vi "Terminal-GearSystem-Getter.vi"(8 "error in (no error)":errorcluster caption="错误输入（无错误）", 11 "read operation timeout (ms)":i32=5000 caption="读操作超时（5000毫秒）") -> (0 "error out":errorcluster caption="错误输出", 3 "设备信息":T1)   [LabVIEW 2014]
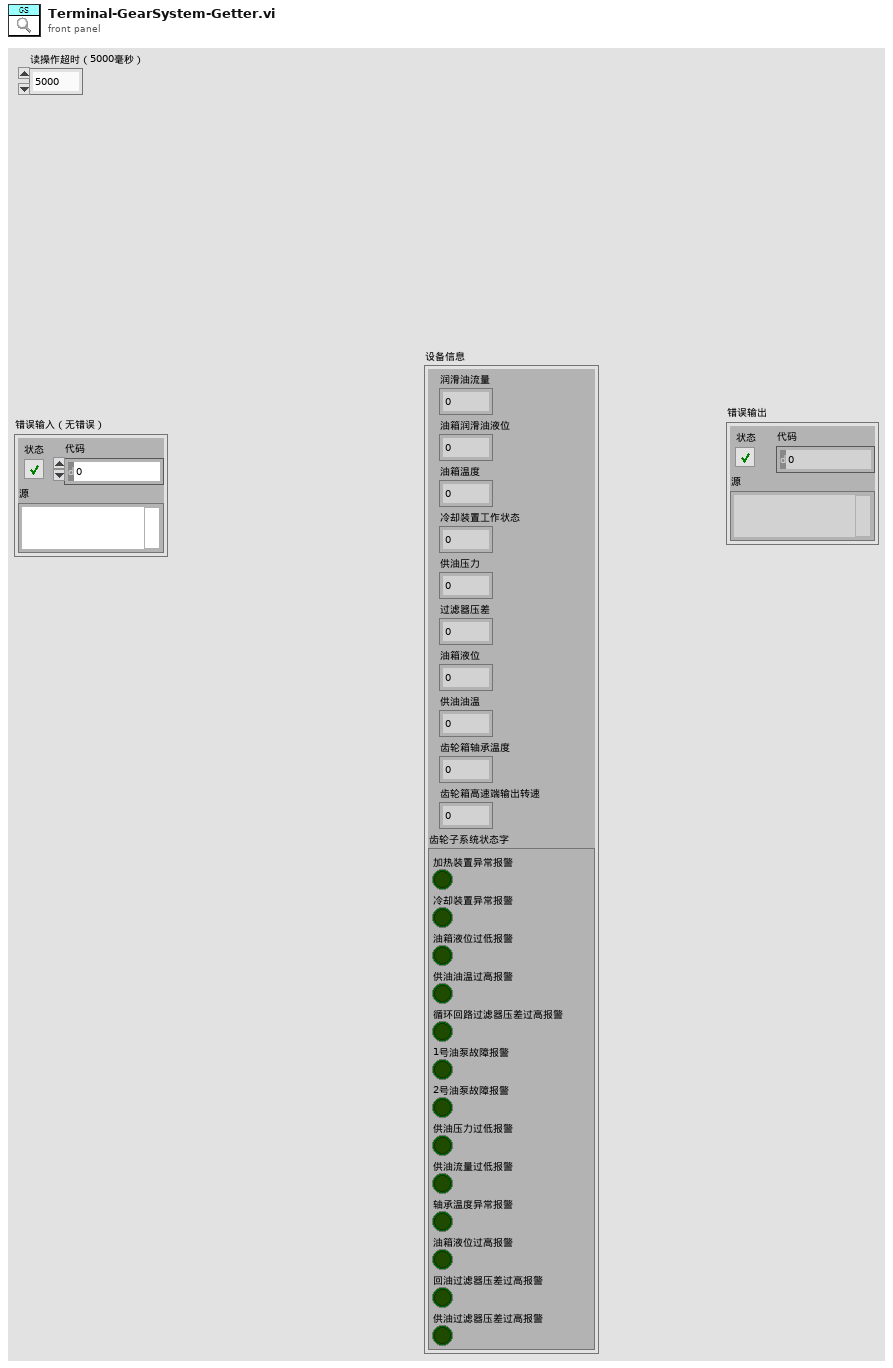
[diagram p1: front panel]
types:
  T1 = cluster{"润滑油流量":u16, "油箱润滑油液位":u16, "油箱温度":u16, "冷却装置工作状态":u16, "供油压力":u16, "过滤器压差":u16, "油箱液位":u16, "供油油温":u16, "齿轮箱轴承温度":u16, "齿轮箱高速端输出转速":u16, "齿轮子系统状态字":cluster{"加热装置异常报警":bool, "冷却装置异常报警":bool, "油箱液位过低报警":bool, "供油油温过高报警":bool, "循环回路过滤器压差过高报警":bool, "1号油泵故障报警":bool, "2号油泵故障报警":bool, "供油压力过低报警":bool, "供油流量过低报警":bool, "轴承温度异常报警":bool, "油箱液位过高报警":bool, "回油过滤器压差过高报警":bool, "供油过滤器压差过高报警":bool}}
  T2 = cluster{"加热装置异常报警":bool, "冷却装置异常报警":bool, "油箱液位过高报警":bool, "油箱液位过低报警":bool, "供油油温过高报警":bool, "供油过滤器压差过高报警":bool, "循环回路过滤器压差过高报警":bool, "回油过滤器压差过高报警":bool, "1号油泵故障报警":bool, "2号油泵故障报警":bool, "供油压力过低报警":bool, "供油流量过低报警":bool, "轴承温度异常报警":bool}
  T3 = cluster{"润滑油流量":u16, "油箱润滑油液位":u16, "油箱温度":u16, "冷却装置工作状态":u16, "供油压力":u16, "过滤器压差":u16, "油箱液位":u16, "供油油温":u16, "齿轮箱轴承温度":u16, "齿轮箱高速端输出转速":u16, "齿轮子系统状态字":cluster{"加热装置异常报警":bool, "冷却装置异常报警":bool, "油箱液位过高报警":bool, "油箱液位过低报警":bool, "供油油温过高报警":bool, "供油过滤器压差过高报警":bool, "循环回路过滤器压差过高报警":bool, "回油过滤器压差过高报警":bool, "1号油泵故障报警":bool, "2号油泵故障报警":bool, "供油压力过低报警":bool, "供油流量过低报警":bool, "轴承温度异常报警":bool}}
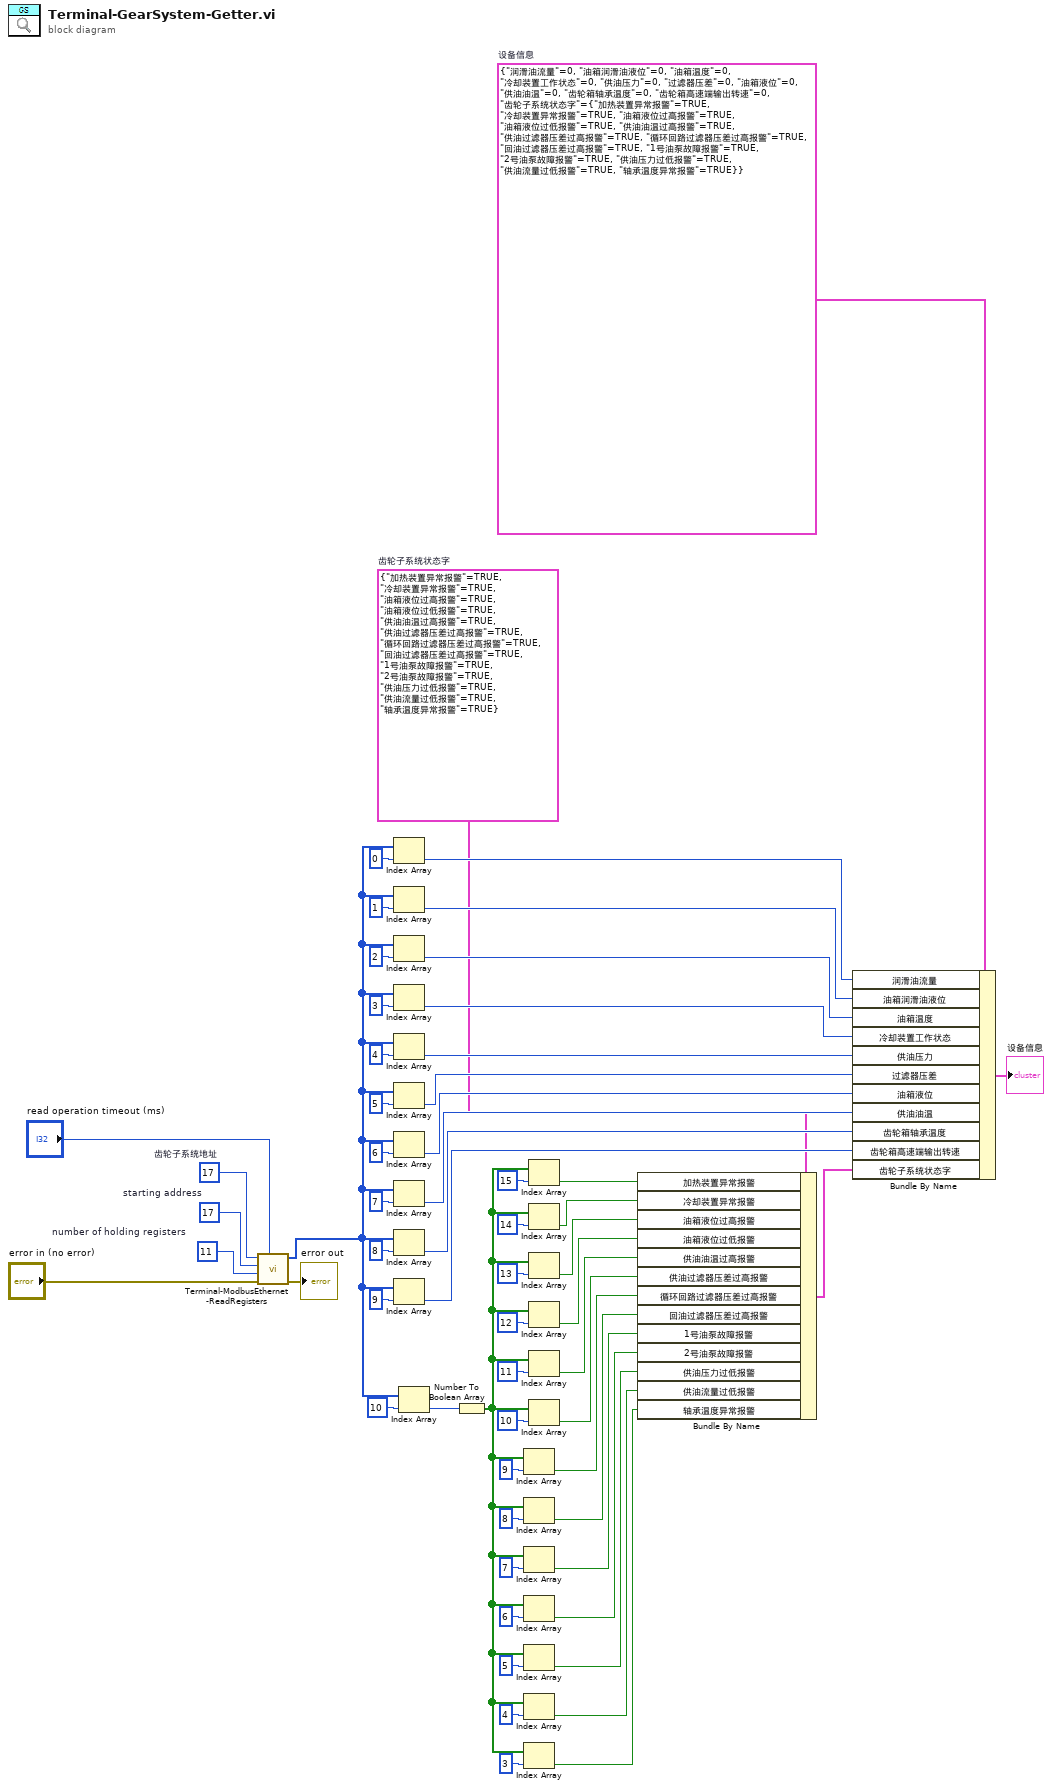
[diagram p0: block diagram]
diagram:
  w23 = T2 {"加热装置异常报警"=TRUE, "冷却装置异常报警"=TRUE, "油箱液位过高报警"=TRUE, "油箱液位过低报警"=TRUE, "供油油温过高报警"=TRUE, "供油过滤器压差过高报警"=TRUE, "循环回路过滤器压差过高报警"=TRUE, "回油过滤器压差过高报警"=TRUE, "1号油泵故障报警"=TRUE, "2号油泵故障报警"=TRUE, "供油压力过低报警"=TRUE, "供油流量过低报警"=TRUE, "轴承温度异常报警"=TRUE}  # 齿轮子系统状态字
  w54 = T3 {"润滑油流量"=0, "油箱润滑油液位"=0, "油箱温度"=0, "冷却装置工作状态"=0, "供油压力"=0, "过滤器压差"=0, "油箱液位"=0, "供油油温"=0, "齿轮箱轴承温度"=0, "齿轮箱高速端输出转速"=0, "齿轮子系统状态字"={"加热装置异常报警"=TRUE, "冷却装置异常报警"=TRUE, "油箱液位过高报警"=TRUE, "油箱液位过低报警"=TRUE, "供油油温过高报警"=TRUE, "供油过滤器压差过高报警"=TRUE, "循环回路过滤器压差过高报警"=TRUE, "回油过滤器压差过高报警"=TRUE, "1号油泵故障报警"=TRUE, "2号油泵故障报警"=TRUE, "供油压力过低报警"=TRUE, "供油流量过低报警"=TRUE, "轴承温度异常报警"=TRUE}}  # 设备信息
  w58 = u16 11  # number of holding registers
  w59 = u16 17  # starting address
  w60 = u8 17  # 齿轮子系统地址
  n1 = call "Terminal-ModbusEthernet-ReadRegisters.vi"("read operation timeout (ms)"="read operation timeout (ms)", "error in"="error in (no error)", "number of holding registers"=w58, "starting address"=w59, "unit ID"=w60) -> ("error out"=→"error out":errorcluster, "register values"=w30:u16[])  [unwired: 5 in]
  n2 = Index Array(array=w30, index=0 ("索引")) -> (element=w52:u16)
  n3 = Index Array(array=w30, index=1 ("索引")) -> (element=w47:u16)
  n4 = Index Array(array=w30, index=2 ("索引")) -> (element=w46:u16)
  n5 = Index Array(array=w30, index=3 ("索引")) -> (element=w45:u16)
  n6 = Index Array(array=w30, index=4 ("索引")) -> (element=w29:u16)
  n7 = Index Array(array=w30, index=5 ("索引")) -> (element=w28:u16)
  n8 = Index Array(array=w30, index=6 ("索引")) -> (element=w27:u16)
  n9 = Index Array(array=w30, index=7 ("索引")) -> (element=w26:u16)
  n10 = Index Array(array=w30, index=8 ("索引")) -> (element=w25:u16)
  n11 = Index Array(array=w30, index=9 ("索引")) -> (element=w24:u16)
  n12 = Index Array(array=w30, index=10 ("索引")) -> (element=w44:u16)
  n13 = Number To Boolean Array(number=w44) -> (Boolean array=w14:bool[])
  n14 = Index Array(array=w14, index=9 ("索引")) -> (element=w7:bool)
  n15 = Index Array(array=w14, index=8 ("索引")) -> (element=w6:bool)
  n16 = Index Array(array=w14, index=7 ("索引")) -> (element=w5:bool)
  n17 = Index Array(array=w14, index=6 ("索引")) -> (element=w4:bool)
  n18 = Index Array(array=w14, index=5 ("索引")) -> (element=w1:bool)
  n19 = Index Array(array=w14, index=4 ("索引")) -> (element=w2:bool)
  n20 = Index Array(array=w14, index=3 ("索引")) -> (element=w3:bool)
  n21 = Index Array(array=w14, index=15 ("索引")) -> (element=w39:bool)
  n22 = Index Array(array=w14, index=14 ("索引")) -> (element=w38:bool)
  n23 = Index Array(array=w14, index=13 ("索引")) -> (element=w37:bool)
  n24 = Index Array(array=w14, index=12 ("索引")) -> (element=w10:bool)
  n25 = Index Array(array=w14, index=11 ("索引")) -> (element=w9:bool)
  n26 = Index Array(array=w14, index=10 ("索引")) -> (element=w8:bool)
  n27 = Bundle By Name(cluster=w23, "加热装置异常报警"=w39, "冷却装置异常报警"=w38, "油箱液位过高报警"=w37, "油箱液位过低报警"=w10, "供油油温过高报警"=w9, "供油过滤器压差过高报警"=w8, "循环回路过滤器压差过高报警"=w7, "回油过滤器压差过高报警"=w6, "1号油泵故障报警"=w5, "2号油泵故障报警"=w4, "供油压力过低报警"=w1, "供油流量过低报警"=w2, "轴承温度异常报警"=w3) -> (w22:T2)
  n28 = Bundle By Name(cluster=w54, "润滑油流量"=w52, "油箱润滑油液位"=w47, "油箱温度"=w46, "冷却装置工作状态"=w45, "供油压力"=w29, "过滤器压差"=w28, "油箱液位"=w27, "供油油温"=w26, "齿轮箱轴承温度"=w25, "齿轮箱高速端输出转速"=w24, "齿轮子系统状态字"=w22) -> (→"设备信息":T3)
